vi "PCO_SetFlimImageProcessingFlow.vi"(0 "ph":u64, 5 "wAsymmetryCorrection":u16(ring) items=["OFF", "ON"], 7 "wOutputMode":u16(ring) items=["normal", "multiply x2"], 11 "error in (no error)":errorcluster {"code" format="%x"}) -> (4 "ph out":u64, 6 "ErrorMessage":i32 format="%x", 15 "error out":errorcluster {"code" format="%x"})   [LabVIEW 2019, in "SDK.lvlib" / "SpecialCommandsFlim.lvlib"]
doc: "<b>Description:</b>\nConfigure parameters of pco.flim specific internal image processing inside the camera. A PCO_ArmCamera command is required to update these settings.\n\n<b>Supported camera type:</b>\npco.flim\n\n<b>Descriptor dependency:</b>\nNone"
uses:
  SpecialCommandsFlim.lvlib
panel:
  in  "wThresholdHigh":u16
  in  "wThresholdLow":u16
  in  "wReferencingMode":u16
  in  "wCalculationMode":u16
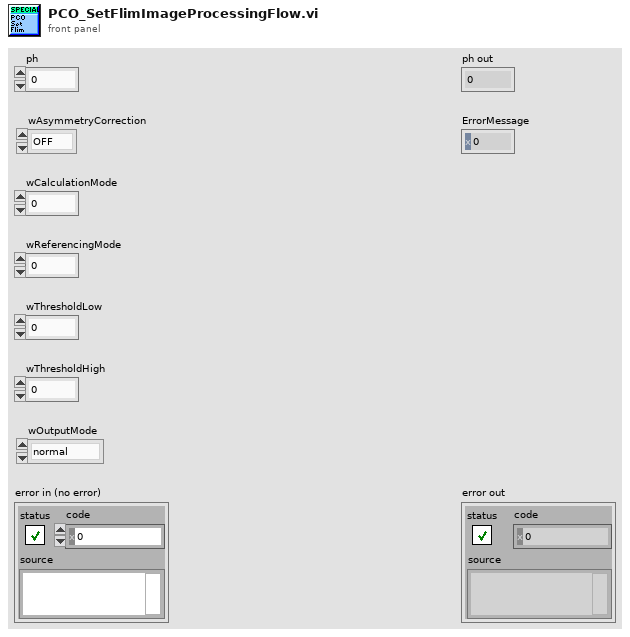
[diagram p1: front panel]
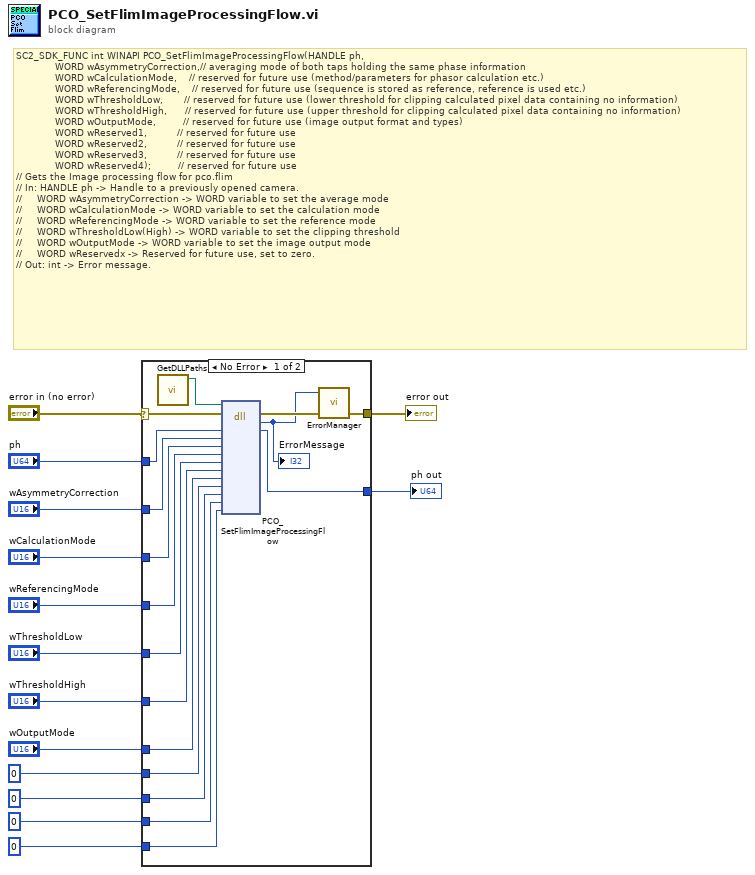
[diagram p0: block diagram]
diagram:
  # "SC2_SDK_FUNC int WINAPI PCO_SetFlimImageProcessingFlow(HANDLE ph, \n             WORD wAsymmetryCorrection,// averaging mode of both taps holding the same phase information\n             WORD wCalculationMode,    // reserved for future use (method/parameters for phasor calculation etc.)\n             WORD wReferencingMode,    // reserved for future use (sequence is stored as reference, reference is used etc.)\n             WORD wThresholdLow,       // reserved for future use (lower threshold for clipping calculated pixel data containing no information)\n             WORD wThresholdHigh,      // reserved for future use (upper threshold for clipping calculated pixel data containing no information)\n             WORD wOutputMode,         // reserved for future use (image output format and types)\n             WORD wReserved1,          // reserved for future use\n             WORD wReserved2,          // reserved for future use\n             WORD wReserved3,          // reserved for future use\n             WORD wReserved4);         // reserved for future use\n// Gets the Image processing flow for pco.flim\n// In: HANDLE ph -> Handle to a previously opened camera.\n//     WORD wAsymmetryCorrection -> WORD variable to set the average mode\n//     WORD wCalculationMode -> WORD variable to set the calculation mode\n//     WORD wReferencingMode -> WORD variable to set the reference mode\n//     WORD wThresholdLow(High) -> WORD variable to set the clipping threshold\n//     WORD wOutputMode -> WORD variable to set the image output mode\n//     WORD wReservedx -> Reserved for future use, set to zero.\n// Out: int -> Error message."
  n1 = case shown="No Error" "error in (no error)" {
    selector: "error in (no error)" -> [w19 w33]
    tunnel: "ph" -> [w31 w32]
    tunnel: [w30 w32] -> w13
    tunnel: "wAsymmetryCorrection" -> [w29 _]
    tunnel: "wCalculationMode" -> [w28 _]
    tunnel: "wReferencingMode" -> [w27 _]
    tunnel: "wThresholdLow" -> [w26 _]
    tunnel: "wThresholdHigh" -> [w25 _]
    tunnel: "wOutputMode" -> [w24 _]
    tunnel: [w18 w33] -> w6
    tunnel: u16 0 ("wReserved1") -> [w23 _]
    tunnel: u16 0 ("wReserved1") -> [w22 _]
    tunnel: u16 0 ("wReserved1") -> [w21 _]
    tunnel: u16 0 ("wReserved1") -> [w20 _]
    frame No Error {
      n2 = call "GetDLLPaths.vi"() -> ("SC2_Cam_Path"=w15:path)  [unwired: 8 in, 3 out]
      n3 = dll-call lib="?" fn="PCO_SetFlimImageProcessingFlow"(path in=w15, error in=w19, "ph"=w31, "wAsymmetryCorrection"=w29, "wCalculationMode"=w28, "wReferencingMode"=w27, "wThresholdLow"=w26, "wThresholdHigh"=w25, "wOutputMode"=w24, "wReserved1"=w23, "wReserved2"=w22, "wReserved3"=w21, "wReserved4"=w20) -> (error out=w17:errorcluster, "return type"=w16:i32, "ph"=w30:u64)  [unwired: 11 in, 1 out]
      "ErrorMessage" <- w16
      n4 = call "ErrorManager.vi"("error in (no error)"=w17, "error code"=w16) -> ("error out"=w18:errorcluster)  [unwired: 2 in, 1 out]
    }
    frame Error {
    }
  }
  "ph out" <- w13
  "error out" <- w6
